vi "Set View.vi"(8 "error in (no error)":errorcluster, 11 "View Selection":T1) -> (0 "error out":errorcluster)   [LabVIEW 2015, in "Main Controller Actor API.lvclass"]
uses:
  Main Controller Actor API.lvclass
  Actor/View.ctl
  Re-use Libraries/Minimal Actor Framework/Messaging/Message/Message.lvclass/Message.ctl
  Globals.vi
  Re-use Libraries/Minimal Actor Framework/Messaging/Message/Message.lvclass
  Actor/Main Controller Actor.lvclass
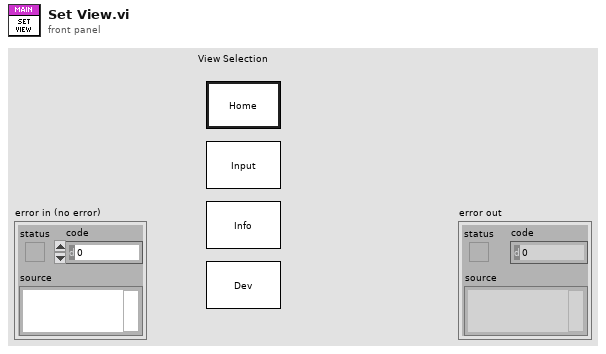
[diagram p1: front panel]
types:
  T1 = typedef "Main Controller Actor.lvclass/View.ctl" = enum32{"Main", "Boolean", "Info", "Dev"}
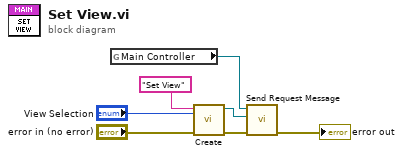
[diagram p0: block diagram]
diagram:
  n1 = global read "Globals.vi" "Main Controller"() -> (w1:refnum<class "Main Controller Actor API.lvclass">)
  n2 = call "Create.vi"("error in (no error)"="error in (no error)", "Data"="View Selection", "Name"="Set View" ("Parameter")) -> ("error out"=w2:errorcluster, "Message out"=w3:refnum<class "Message.lvclass">)  [unwired: 7 in]
  n3 = call-dynamic "Send Request Message.vi"("error in (no error)"=w2, "Message"=w3, "Actor API in"=w1) -> ("error out"=→"error out":errorcluster)  [unwired: 8 in]
